vi "Audio Collect.vi"() -> ()   [LabVIEW 2013]
uses:
  <vilib>/DAQmx/read.llb/DAQmx Read.vi
  <vilib>/DAQmx/read.llb/DAQmx Read (Analog 1D Wfm NChan NSamp).vi
  <vilib>/DAQmx/miscellaneous.llb/DAQmx Fill In Error Info.vi
panel:
  out "data":waveform(dbl)[](graph)
  in  "stop":bool
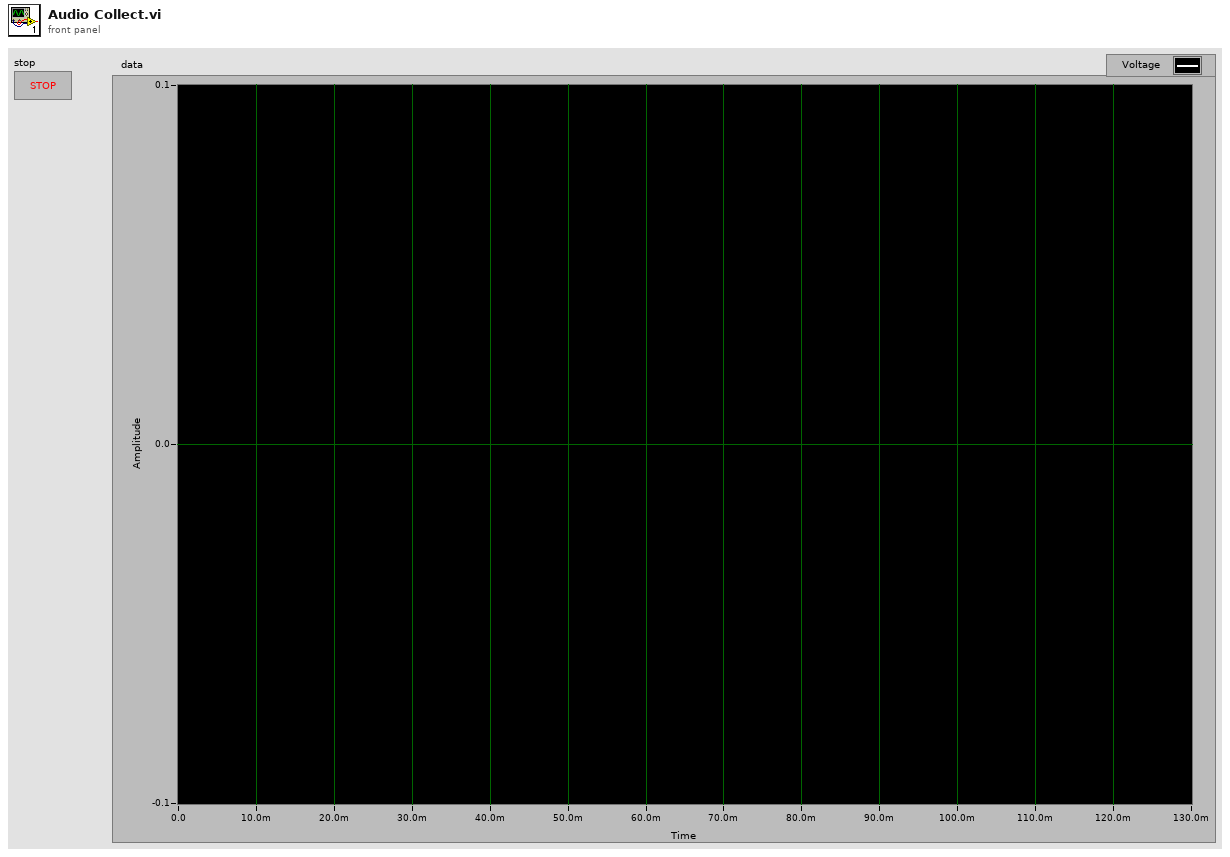
[diagram p1: front panel]
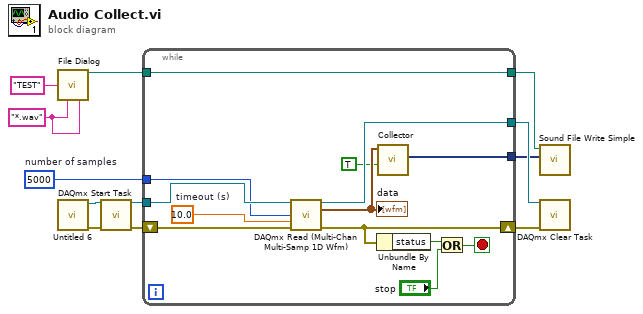
[diagram p0: block diagram]
diagram:
  w4 = "*.wav" ("pattern label")
  w8 = 5000  # number of samples
  n1 = call "File Dialog"("default name"="TEST", "pattern (all files)"=w4, "pattern label"=w4) -> ("selected path"=w5:path)  [unwired: 9 in, 3 out]
  n2 = call "Untitled 6.vi"() -> ("error out"=w12:errorcluster, "task out"=w11:refnum<k21>)  [unwired: 10 in]
  n3 = call <vilib>:"DAQmx Start Task.vi"("task/channels in"=w11, "error in"=w12) -> ("task out"=w6:refnum<k21>, "error out"=w7:errorcluster)  [unwired: 12 in]
  n4 = while {
    tunnel: w6 -> [w25]
    tunnel: w8 -> [w22]
    tunnel: [w23] -> w10
    shift-right: [w20] -> w9
    shift-left: w7 -> [w24]
    tunnel: w5 -> [w14]
    tunnel: [w15] -> w2
    tunnel: [w14] -> w1
    stop <- w19 stop-if-true
    w17 = 10.0  # timeout (s)
    n5 = call-poly "DAQmx Read (Multi-Chan Multi-Samp 1D Wfm).vi"("task/channels in"=w25, "number of samples per channel"=w22, "timeout"=w17, "error in"=w24) -> ("task out"=w23:refnum<k21>, "data"=w16:waveform(dbl)[], "error out"=w20:errorcluster)  [unwired: 9 in]
    "data" <- w16
    n6 = Unbundle By Name(w20) -> ("status"=w21:bool)
    n7 = call "Collector"("Enable"=TRUE, "Signals"=w16) -> ("Collected Signals"=w15:dynamicdata)  [unwired: 8 in, 1 out]
    n8 = Or(x=w21, y="stop") -> (x .or. y?=w19:bool)
  }
  n9 = call <vilib>:"Sound File Write Simple.vi"("data"=w2, "path"=w1) -> ()  [unwired: 8 in, 2 out]
  n10 = call <vilib>:"DAQmx Clear Task.vi"("task in"=w10, "error in"=w9) -> ()  [unwired: 13 in, 1 out]
